vi "Write timeout ms.vi"(8 "error in (no error)":errorcluster, 10 "timeout ms":i32=1000, 11 "Event_Syslog in":refnum<class "Event_Syslog.lvclass">) -> (0 "error out":errorcluster, 3 "Event_Syslog out":refnum<class "Event_Syslog.lvclass">)   [LabVIEW 2021, in "Event_Syslog.lvclass"]
uses:
  Event_Syslog.lvclass
  Event_Syslog.lvclass/Event_Syslog.ctl
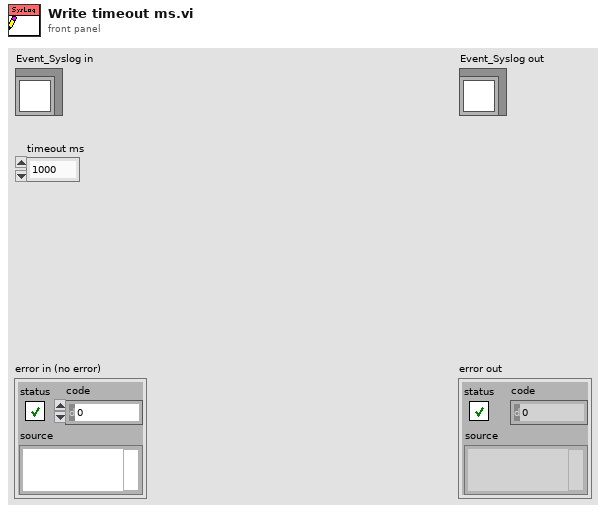
[diagram p1: front panel]
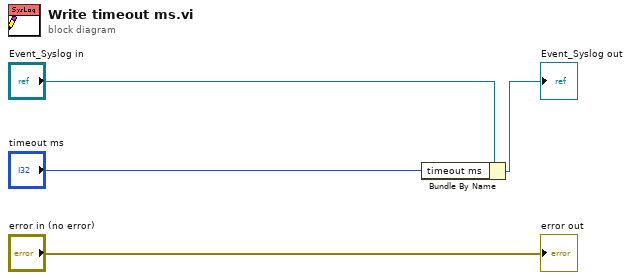
[diagram p0: block diagram]
diagram:
  n1 = Bundle By Name(cluster="Event_Syslog in", "timeout ms"="timeout ms") -> (→"Event_Syslog out":refnum<class "Event_Syslog.lvclass">)
  "error out" <- "error in (no error)"
